vi "FilterMetrics.vi"(11 "supported metrics":string[](array[string])) -> (3 "supported 60s metrics":string[](array[string]))   [LabVIEW 2017, in "McsaAnalysisLowUpdate.lvlib"]
uses:
  <vilib>/addons/InsightCM/Devices/Shared/Mcsa/McsaAnalysisLowUpdate/McsaAnalysisLowUpdate.lvlib
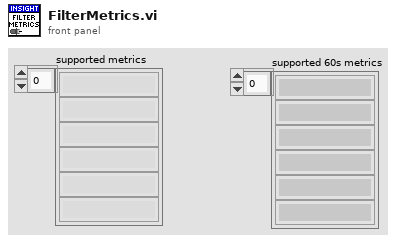
[diagram p1: front panel]
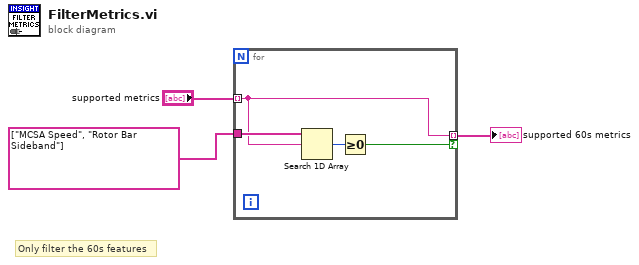
[diagram p0: block diagram]
diagram:
  # "Only filter the 60s features"
  n1 = for {
    tunnel: "supported metrics" -> [w5] mode=indexing
    tunnel: string[] ["MCSA Speed", "Rotor Bar Sideband"] ("value") -> [w7]
    tunnel: [w5] -> w1 mode=indexing if=w4
    n2 = Search 1D Array(1D array=w7, element=w5) -> (index of element=w6:i32)  [unwired: 1 in]
    n3 = Greater Or Equal To 0?(x=w6) -> (x >= 0?=w4:bool)
  }
  "supported 60s metrics" <- w1
